vi "Add Error Functional Global.vi"(8 "Error In":errorcluster) -> (0 "Error Out":errorcluster)   [LabVIEW 2012, in "OpenCLV x64.lvlib"]
doc: "Add any type of Labview error for logging. When an error is added, the time, location, and type of error are logged and can be viewed by calling <b>View Error</b> found in the same polymorphic VI as <b>Add Error</b>.\n\nBy default, when an error is logged, a pop-up occurs that displays the log information. These pop-ups can be supressed by calling <b>Quite Mode</b> or re-enabled by calling <b>Verbose Mode</b>, both found in the same polymorphic VI as <b>Add Error</b>"
uses:
  OpenCLV x64.lvlib
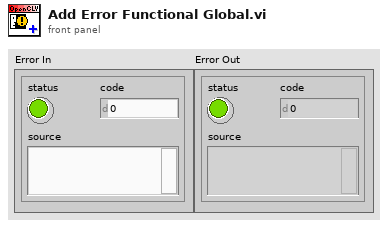
[diagram p1: front panel]
types:
  T1 = enum16{"Initialize", "Add Error", "View Error Log", "Save Error Log", "Set Verbose Mode", "Set Quite Mode"}
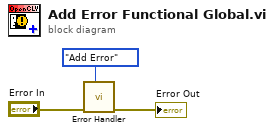
[diagram p0: block diagram]
diagram:
  n1 = call "Error Handler.vi"("Error Handler States"=T1."Add Error", "Error In"="Error In") -> ("Error Out"=→"Error Out":errorcluster)  [unwired: 9 in]
